vi "Obliczanie wzmocnienia Global.vi"() -> ()   [LabVIEW 2014]
panel:
  in  "b34":dbl
  in  "a34":dbl
  in  "b12":dbl
  in  "a12":dbl
  in  "b4":dbl
  in  "a4":dbl
  in  "b3":dbl
  in  "a3":dbl
  in  "b2":dbl=-5.0
  in  "b1":dbl=1.0
  in  "a2":dbl=0.75
  in  "a1":dbl=4.0
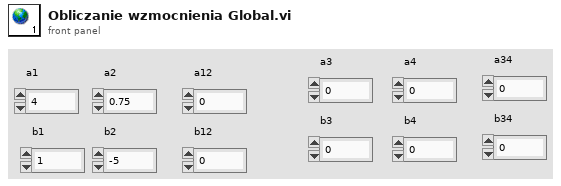
[diagram p1: front panel]
diagram:
